vi "BinF_SaveHeader.vi"(7 "BinF File Settings":T1={"Version"=2, "Data Representation"=enum."I16", "# columns (samples per channel)"=300, "# rows (channels)"=150, "# pre-trigger samples"=20, "Sample rate"=1000.0, "ADC offset"=256.0, "Scale factor"=0.001}, 8 "error in":errorcluster, 11 "refnum":refnum<file>) -> (0 "error out":errorcluster, 3 "refnum out":refnum<file>)   [LabVIEW 2015]
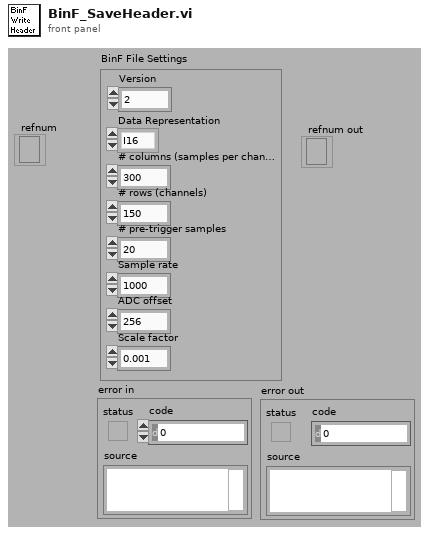
[diagram p1: front panel]
types:
  T1 = cluster{"Version":i16, "Data Representation":enum16{"Undefined", "I8", "I16", "I32", "I64", "U8", "U16", "U32", "U64", "SGL", "DBL", "EXT"}, "# columns (samples per channel)":i64, "# rows (channels)":i64, "# pre-trigger samples":i64, "Sample rate":dbl, "ADC offset":dbl, "Scale factor":dbl}
  T2 = enum16{"Undefined", "I8", "I16", "I32", "I64", "U8", "U16", "U32", "U64", "SGL", "DBL", "EXT"}
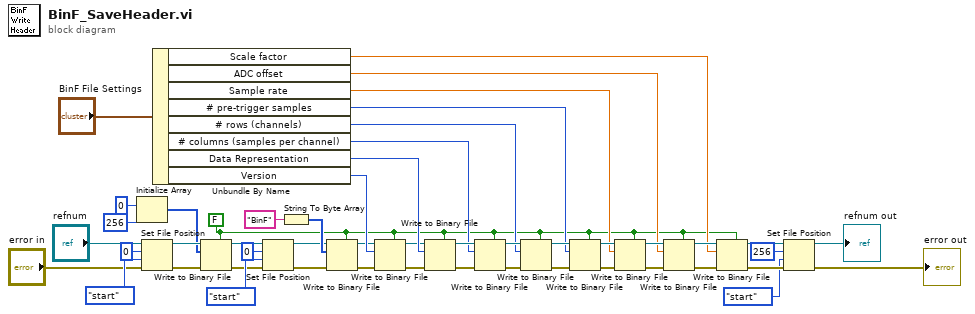
[diagram p0: block diagram]
diagram:
  w1 = FALSE ("prepend array or string size? (T)")
  n1 = Initialize Array(u8 0 ("element"), 256 ("dimension size")) -> (w21:u8[])
  n2 = Set File Position(offset (in bytes) (0)=i64 0, refnum="refnum", from (0:start)=enum16{"start", "end", "current"}."start", error in="error in") -> (refnum out=w25:refnum<file>, error out=w24:errorcluster)
  n3 = Unbundle By Name("BinF File Settings") -> ("Scale factor"=w6:dbl, "ADC offset"=w7:dbl, "Sample rate"=w8:dbl, "# pre-trigger samples"=w9:i64, "# rows (channels)"=w10:i64, "# columns (samples per channel)"=w11:i64, "Data Representation"=w12:T2, "Version"=w4:i16)
  n4 = Write to Binary File(file (use dialog)=w25, data=w21, error in=w24, 5:w1) -> (refnum out=w26:refnum<file>, error out=w27:errorcluster)  [unwired: 2 in, 1 out]
  n5 = Set File Position(offset (in bytes) (0)=i64 0, refnum=w26, from (0:start)=enum16{"start", "end", "current"}."start", error in=w27) -> (refnum out=w44:refnum<file>, error out=w45:errorcluster)
  n6 = String To Byte Array(string="BinF") -> (unsigned byte array=w47:u8[])
  n7 = Write to Binary File(file (use dialog)=w44, data=w47, error in=w45, 5:w1) -> (refnum out=w3:refnum<file>, error out=w46:errorcluster)  [unwired: 2 in, 1 out]
  n8 = Write to Binary File(file (use dialog)=w3, data=w4, error in=w46, 5:w1) -> (refnum out=w2:refnum<file>, error out=w5:errorcluster)  [unwired: 2 in, 1 out]
  n9 = Write to Binary File(file (use dialog)=w2, data=w12, error in=w5, 5:w1) -> (refnum out=w41:refnum<file>, error out=w40:errorcluster)  [unwired: 2 in, 1 out]
  n10 = Write to Binary File(file (use dialog)=w41, data=w11, error in=w40, 5:w1) -> (refnum out=w38:refnum<file>, error out=w39:errorcluster)  [unwired: 2 in, 1 out]
  n11 = Write to Binary File(file (use dialog)=w38, data=w10, error in=w39, 5:w1) -> (refnum out=w36:refnum<file>, error out=w37:errorcluster)  [unwired: 2 in, 1 out]
  n12 = Write to Binary File(file (use dialog)=w36, data=w9, error in=w37, 5:w1) -> (refnum out=w34:refnum<file>, error out=w35:errorcluster)  [unwired: 2 in, 1 out]
  n13 = Write to Binary File(file (use dialog)=w34, data=w8, error in=w35, 5:w1) -> (refnum out=w32:refnum<file>, error out=w33:errorcluster)  [unwired: 2 in, 1 out]
  n14 = Write to Binary File(file (use dialog)=w32, data=w7, error in=w33, 5:w1) -> (refnum out=w19:refnum<file>, error out=w20:errorcluster)  [unwired: 2 in, 1 out]
  n15 = Write to Binary File(file (use dialog)=w19, data=w6, error in=w20, 5:w1) -> (refnum out=w16:refnum<file>, error out=→"error out":errorcluster)  [unwired: 2 in, 1 out]
  n16 = Set File Position(offset (in bytes) (0)=i64 256, refnum=w16, from (0:start)=enum16{"start", "end", "current"}."start") -> (refnum out=→"refnum out":refnum<file>)  [unwired: 1 in, 1 out]
